vi "First_Program.vi"() -> ()   [LabVIEW 2012]
uses:
  Code/Control 1.ctl
  SubVIs/LVPresent_Globals.vi
  BotSpeakSubs/BotspeakSettingsUsed.vi
panel:
  in  "State":T1
  in  "Open":bool
  in  "Port":u8=13
  in  "Run":bool
  # "Writing LabVIEW Code\n\nPush the Run button - does the light built into the board turn on?  Change it from LO to HI - and run it again.  What happens? Try changing the Port - from pin 13 to pin 5. Note that the LO/HI states of the RGB LEDs is the opposite of the on-board LEDs. This is called a LabVIEW diagram - it is where your program resides - this program is simple - it changes the state of pin 13.  Once you open the program (click \"Open\") try clicking on the diagram, moving things around and see if you can break things."
  # "Click the open button to open the program and see more helpful tips!"
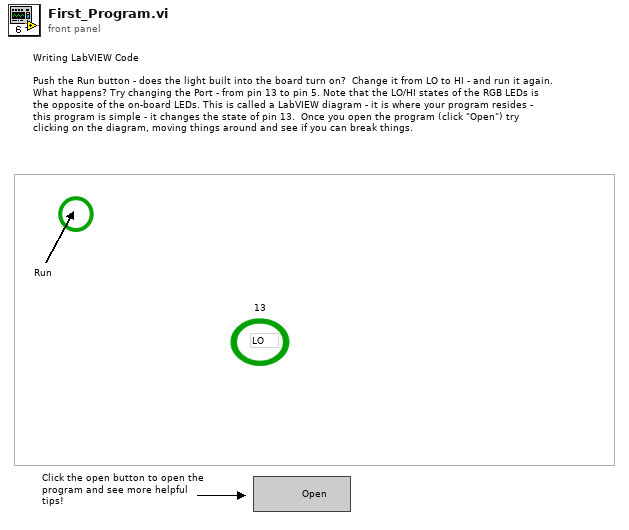
[diagram p1: front panel]
types:
  T1 = typedef "Control 1.ctl" = enum16{"LO", "HI"}
  T2 = typedef "BotSpeak_Control.ctl" = cluster{"Address":string, "Reply EOF":string, "Hardware":string, "Retries":i8, "Timeout":i32}
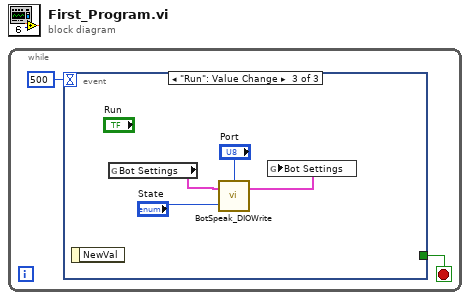
[diagram p0: block diagram]
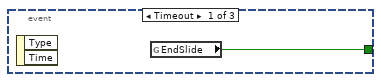
[diagram p2: hidden frame]
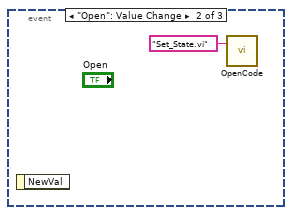
[diagram p3: hidden frame]
diagram:
  n1 = while {
    stop <- w2 stop-if-true
    n2 = event shown="[2] \"Run\": Value Change" {
      selector: _ -> [_ _ _]
      dyn-events: _ -> [_ _ _]
      timeout: 500 -> [_ _ _]
      tunnel: [w3 _ _] -> w2
      event Timeout {
        n3 = event-data() -> ()  [unwired: 1 in, 2 out]
        n4 = global read "LVPresent_Globals.vi" "EndSlide"() -> (w3:bool)
      }
      event "Open": Value Change {
        n5 = event-data() -> ()  [unwired: 1 in, 1 out]
        n6 = call "OpenCode.vi"("Code name"="Set_State.vi") -> ()  [unwired: 3 in]
      }
      event "Run": Value Change {
        n7 = event-data() -> ()  [unwired: 1 in, 1 out]
        n8 = global read "BotspeakSettingsUsed.vi" "Bot Settings"() -> (w6:T2)
        n9 = call <userlib>:"BotSpeak_DIOWrite.vi"("State"="State", "Bot Settings"=w6, "DIO Line"="Port") -> ("Bot Settings"=w5:T2)  [unwired: 1 out]
        n10 = global write "BotspeakSettingsUsed.vi" "Bot Settings"(w5) -> ()
      }
    }
  }
